vi "Get CGRAM Address by Index.vi"(7 "self defined pattern":enum16{"5 X 10", "5 X 8"}(ring)=enum."5 X 8", 10 "index of row":u8 format="%.0b", 11 "customized character index":u8) -> (3 "CGRAM address":u8 format="%.0b")   [LabVIEW 2017, in "HD44780.lvclass"]
uses:
  HD44780.lvclass
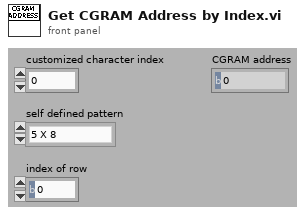
[diagram p1: front panel]
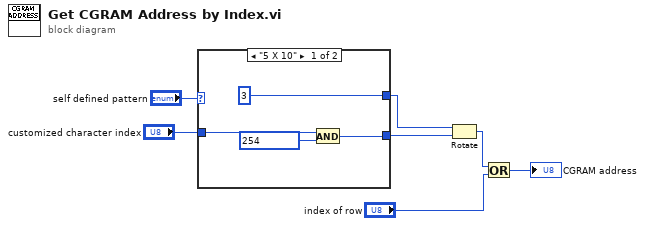
[diagram p0: block diagram]
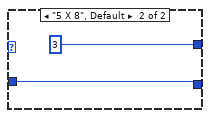
[diagram p2: hidden frame]
diagram:
  n1 = case shown="\"5 X 10\"" "self defined pattern" {
    tunnel: [i16 3 ("y") i16 3 ("y")] -> w4
    tunnel: "customized character index" -> [w10 w12]
    tunnel: [w8 w12] -> w1
    frame "5 X 10" {
      n2 = And(x=w10, y=u8 254) -> (x .and. y?=w8:u8)
    }
    frame "5 X 8", Default {
    }
  }
  n3 = Rotate(1:w1, 2:w4) -> (0:w7:u8)
  n4 = Or(x=w7, y="index of row") -> (x .or. y?=→"CGRAM address":u8)
